vi "Galil.vi"() -> ()   [LabVIEW 2010]
panel:
  in  "Galil.IGalil":refnum<k7>
  out "MG TIME":string
  out "Library Version:":string
  out "error out":errorcluster
  out "Connected To:":string
  in  "Connection String":string
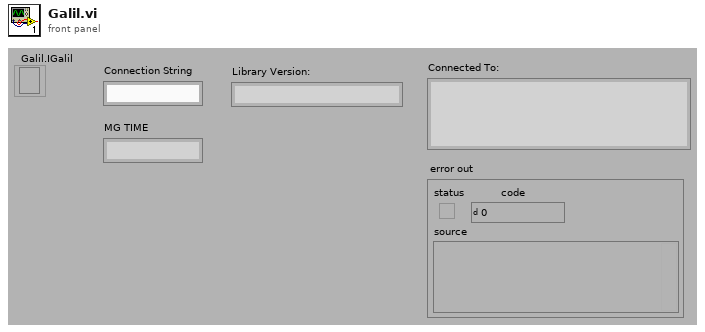
[diagram p1: front panel]
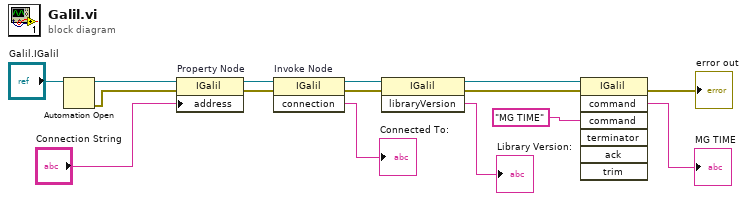
[diagram p0: block diagram]
diagram:
  n1 = Automation Open(Automation Refnum="Galil.IGalil") -> (Automation Refnum=w15:refnum<k7>, error out=w12:errorcluster)  [unwired: 1 in, 2 out]
  n2 = property on="Property Node" class="IGalil"(reference=w15, error in=w12, "address"="Connection String") -> (reference out=w14:refnum<k7>, error out=w13:errorcluster)
  n3 = invoke on="Invoke Node" class="IGalil" method="connection"(reference=w14, error in=w13) -> (reference out=w9:refnum<k7>, error out=w8:errorcluster, "connection"=→"Connected To:":string)  [unwired: 1 in]
  n4 = invoke class="IGalil" method="libraryVersion"(reference=w9, error in=w8) -> (reference out=w6:refnum<k7>, error out=w5:errorcluster, "libraryVersion"=→"Library Version:":string)  [unwired: 1 in]
  n5 = invoke class="IGalil" method="command"(reference=w6, error in=w5, "command"="MG TIME") -> (error out=→"error out":errorcluster, "command"=→"MG TIME":string)  [unwired: 4 in, 5 out]
